vi "Write Analogue.vi"(8 "error in (no error)":errorcluster, 10 "Output":bool, 11 "Keysight 6700C in":refnum<class "Keysight 6700C.lvclass">) -> (0 "error out":errorcluster, 3 "Keysight 6700C out":refnum<class "Keysight 6700C.lvclass">)   [LabVIEW 2019, in "Concrete.lvlib" / "Keysight 6700C.lvclass"]
uses:
  Keysight 6700C.lvclass
  Keysight 6700C.lvclass/Keysight 6700C.ctl
  <instrlib>/Agilent N6700/Agilent N6700 Series.lvlib
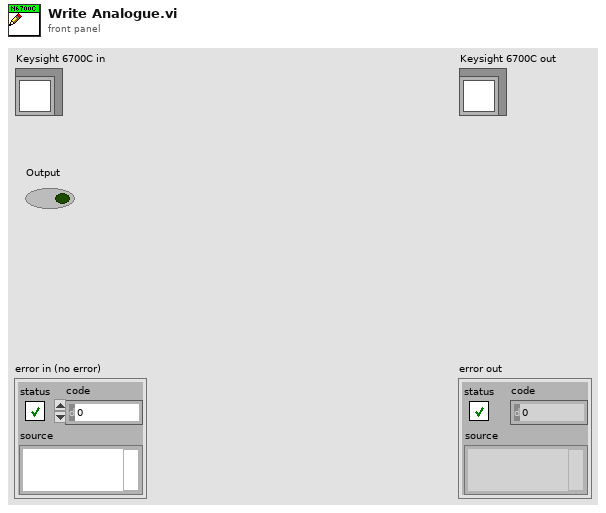
[diagram p1: front panel]
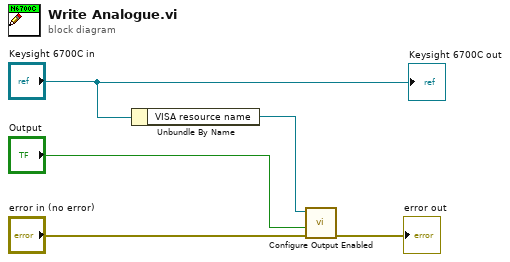
[diagram p0: block diagram]
diagram:
  n1 = Unbundle By Name("Keysight 6700C in") -> ("VISA resource name"=w4:refnum<visa-resource-name>)
  n2 = call <instrlib>:"Configure Output Enabled.vi"("error in (no error)"="error in (no error)", "Enable Output (False)"="Output", "VISA resource name"=w4) -> ("error out"=→"error out":errorcluster)  [unwired: 7 in, 1 out]
  "Keysight 6700C out" <- "Keysight 6700C in"
